vi "Load Plugin From Enum.vi"(4 "error in (no error)":errorcluster, 7 "Plugin Type":T1=enum."Blue") -> (0 "error out":errorcluster, 3 "Generic Plugin.lvclass":refnum<class "Generic Plugin.lvclass">)   [LabVIEW 2019, in "Generic Plugin.lvclass"]
uses:
  Generic Plugin.lvclass
  Plugin Type.ctl
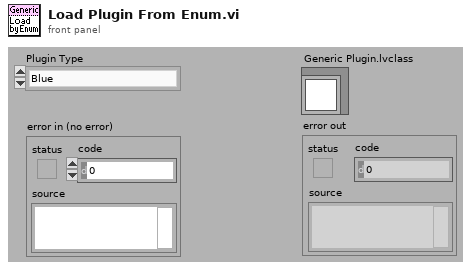
[diagram p1: front panel]
types:
  T1 = typedef "Generic Plugin.lvclass/Plugin Type.ctl" = enum16{"<select plugin>", "Orange", "Blue"}
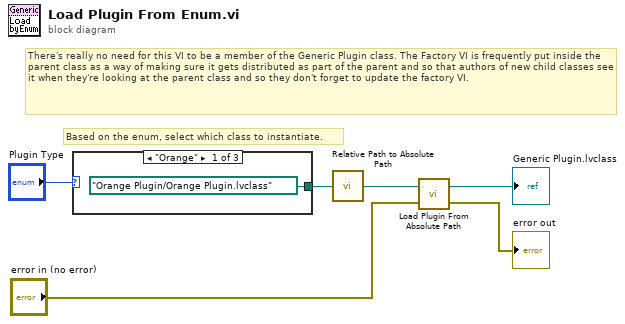
[diagram p0: block diagram]
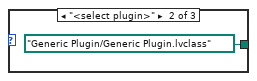
[diagram p2: hidden frame]
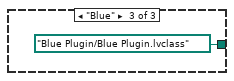
[diagram p3: hidden frame]
diagram:
  # "There's really no need for this VI to be a member of the Generic Plugin class. The Factory VI is frequently put inside the parent class as a way of making sure it gets distributed as part of the parent and so that authors of new child classes see it when they're looking at the parent class and so they don't forget to update the factory VI."
  # "Based on the enum, select which class to instantiate."
  n1 = case shown="\"Orange\"" "Plugin Type" {
    tunnel: [path "Orange Plugin/Orange Plugin.lvclass" path "Generic Plugin/Generic Plugin.lvclass" path "Blue Plugin/Blue Plugin.lvclass"] -> w3
    frame "Orange" {
    }
    frame "<select plugin>" {
    }
    frame "Blue" {
    }
  }
  n2 = call "Relative Path to Absolute Path.vi"("Relative Path"=w3) -> ("Absolute Path"=w2:path)
  n3 = call "Load Plugin From Absolute Path.vi"("error in (no error)"="error in (no error)", "Absolute Path"=w2) -> ("error out"=→"error out":errorcluster, "Generic Plugin.lvclass"=→"Generic Plugin.lvclass":refnum<class "Generic Plugin.lvclass">)
